vi "Start Trace.vi"(7 "Client URI":refnum<class "URI.lvclass">, 10 "error in (no error)":errorcluster) -> (2 "error out":errorcluster, 3 "RequestTraceLog out":refnum<class "RequestTraceLog.lvclass">)   [LabVIEW 2020, in "HTTP Server.lvlib" / "RequestTraceLog.lvclass"]
uses:
  RequestTraceLog.lvclass
  RequestTraceLog.lvclass/RequestTraceLog.ctl
  Trace Item.ctl
  HTTP Server.lvlib
  Processing Step.ctl
  lv-uri/URI/URI/URI.lvclass
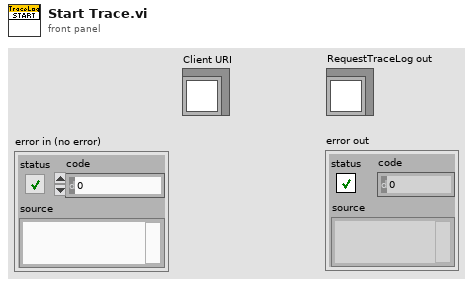
[diagram p1: front panel]
types:
  T1 = typedef "HTTP Server.lvlib/Trace Item.ctl" = cluster{"Duration":dbl, "Step":T2, "Class":string, "Info":string, "Status":bool, "Code":i32, "Time":dbl}
  T2 = typedef "HTTP Server.lvlib/Processing Step.ctl" = enum16{"Connection", "Request", "Routing", "Controller Init", "Controller", "Response", "Complete", "Exception"}
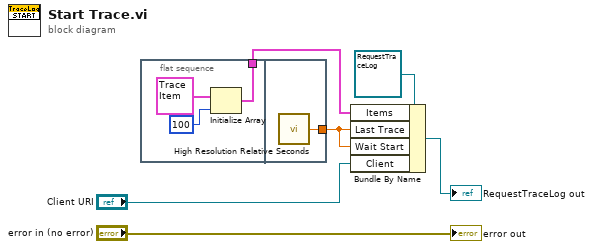
[diagram p0: block diagram]
diagram:
  n1 = flat-sequence {
    tunnel: [w7] -> w3
    tunnel: [w10] -> w2
    frame #0 {
      n2 = Initialize Array(T1 {"Duration"=0.0, "Step"=enum."Connection", "Class"="", "Info"="", "Status"=FALSE, "Code"=0, "Time"=0.0} ("Trace Item"), 100 ("dimension size")) -> (w7:T1[])
    }
    frame #1 {
      n3 = call <vilib>:"High Resolution Relative Seconds.vi"() -> ("relative seconds"=w10:dbl)
    }
  }
  n4 = Bundle By Name(cluster=refnum<class "RequestTraceLog.lvclass"> refnum ("RequestTraceLog in"), "Items"=w3, "Last Trace"=w2, "Wait Start"=w2, "Client"="Client URI") -> (→"RequestTraceLog out":refnum<class "RequestTraceLog.lvclass">)
  "error out" <- "error in (no error)"
